vi "Get SQL formatted value.vi"(8 "error in (no error)":errorcluster, 11 "Numeric Column in":refnum<class "Numeric Column.lvclass">) -> (0 "error out":errorcluster, 2 "Formatted Value":string, 3 "Numeric Column out":refnum<class "Numeric Column.lvclass">)   [LabVIEW 2020, in "Basic Columns.lvlib" / "Numeric Column.lvclass"]
uses:
  Numeric Column.lvclass
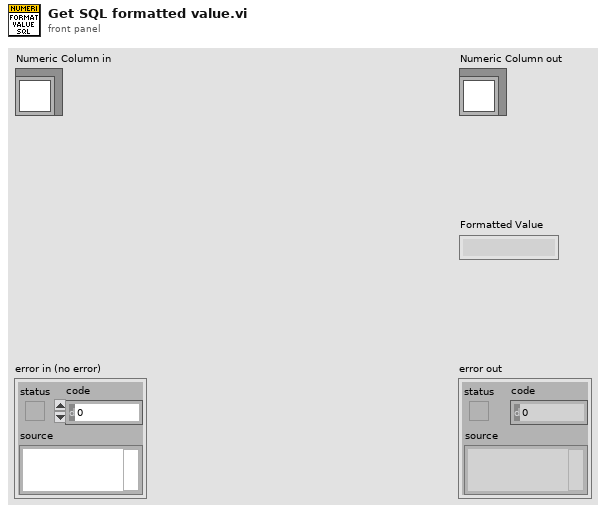
[diagram p1: front panel]
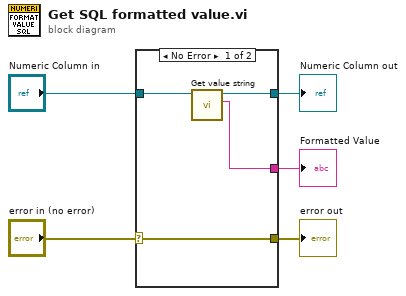
[diagram p0: block diagram]
diagram:
  n1 = case shown="No Error" "error in (no error)" {
    selector: "error in (no error)" -> [w6 w10]
    tunnel: "Numeric Column in" -> [w9 w11]
    tunnel: [w8 w11] -> w3
    tunnel: [w6 w10] -> w2
    tunnel: [w7 _] -> w1
    frame No Error {
      n2 = call-dynamic "Get value string.vi"("Column in"=w9) -> ("Value"=w7:string, "Column out"=w8:refnum<class "Numeric Column.lvclass">)  [unwired: 8 in, 1 out]
    }
    frame Error {
    }
  }
  "error out" <- w2
  "Numeric Column out" <- w3
  "Formatted Value" <- w1
